vi "Measure Jt curve.vi"(4 "Skip pixel?":bool, 6 "Scan settings":T1={"J-V scan"=TRUE, "J-t scan"=FALSE, "Min voltage (V)"=0.0, "Max voltage (V)"=1.4, "Step (V)"=0.01, "Measurement delay (ms)"=10.0, "1st scan FB-SC"=TRUE, "Inverted structure"=FALSE, "Stabilisation time (s)"=0.0, "Stabilisation mode"=0, "Stabilisation value (V or A) "=0.0, "Step time (s)"=1.0, "Integration time"=0, "Repeat light scans"=FALSE, "Stabilisation in the dark?"=FALSE, "J-t Min (V)"=0.0, "J-t Max (V)"=1.4, "J-t Step (V)"=0.01, "Max. power stabilisation"=FALSE, "J-t 1st scan FB-SC"=TRUE, "J-t Inverted structure"=FALSE, "Max power tracking"=FALSE, "Vmp (V)"=0.7, "Total stabilisation time (s)"=100.0, "J-t best pixel only"=0, "Max power best pixel only"=0, "Vmp from J-V scan"=FALSE, "Intensity dependence"=FALSE, "P dep best pixel only"=0, "External quantum efficiency"=FALSE, "EQE best pixel only"=0, "WL min (nm)"=300.0, "WL max (nm)"=900.0, "WL step (nm)"=5.0, "Wait (ms)"=100.0, "No. of repeat scans"=2.0, "Only repeat for best pixel"=0, "Chopper Freq. min (Hz)"=90.0, "Time Constant min (s)"=2.0, "Stabilisation time step (s)"=1.0, "Illumination conditions"=2, "Scan rate min (V/s)"=0.1, "Scan rate max (V/s)"=1.0, "No. of scan rate steps"=1.0, "Scan rate voltage step priority"=FALSE, "Scan rate measurement delay priority"=FALSE, "J-t Illumination conditions"=0, "Chopper Freq. max (Hz)"=200.0, "No. of freq. steps"=1.0, "Time Constant max (s)"=2.0, "No. of t const. steps"=1.0, "White bias min (no. of suns)"=0.1, "White bias max (no. of suns)"=1.0, "No. of white bias steps"=1.0, "Repeat EQE scans"=FALSE, "No. of EQE scans"=2.0, "Max P stab. Specific voltage"=FALSE} {"No. of EQE scans" min=1.0 step=1.0; "No. of white bias steps" min=1.0 step=1.0; "No. of t const. steps" min=1.0 step=1.0; "Time Constant max (s)" items=["0.01s", "0.03s", "0.1s", "0.3s", "1s", "3s"]; "No. of freq. steps" min=1.0 step=1.0; "J-t Illumination conditions" items=["Light only", "Dark only", "Light then dark", "Dark then light"]; "No. of scan rate steps" min=1.0 step=1.0; "Illumination conditions" items=["Light only", "Dark only", "Light then dark", "Dark then light", "Light then dark then light", "Dark then light then dark"]; "Time Constant min (s)" items=["0.01s", "0.03s", "0.1s", "0.3s", "1s", "3s"]; "Only repeat for best pixel" items=["only for best pixel", "for best 2 pixels", "for best 3 pixels", "for best 4 pixels", "for best 5 pixels", "for best 6 pixels", "for best 7 pixels", "for all pixels"]; "No. of repeat scans" min=1.0 step=1.0; "EQE best pixel only" items=["only the best pixel", "the best 2 pixel", "the best 3 pixel", "the best 4 pixel", "the best 5 pixel", "the best 6 pixel", "the best 7 pixel", "all pixels"]; "P dep best pixel only" items=["only the best pixel", "the best 2 pixels", "the best 3 pixels", "the best 4 pixels", "the best 5 pixels", "the best 6 pixels", "the best 7 pixels", "all pixels"]; "Max power best pixel only" items=["only the best pixel", "the best 2 pixels", "the best 3 pixels", "the best 4 pixels", "the best 5 pixels", "the best 6 pixels", "the best 7 pixels", "all pixels"]; "J-t best pixel only" items=["only the best pixel", "the best 2 pixels", "the best 3 pixels", "the best 4 pixels", "the best 5 pixels", "the best 6 pixels", "the best 7 pixels", "all pixels"]; "Integration time" items=["Fast", "Normal", "High Accuracy"]; "Stabilisation mode" items=["V", "I"]; "Measurement delay (ms)" min=10.0}, 7 "Cell details cluster":T3={"Cell Position"=16, "Cell Label"="", "Pixel to measure"=0, "Area (cm^2)"=0.126, "Variable"="", "Variable value"="", "Scan settings in queue"=0, "Light or dark"="", "Measurement Type"=""} {"Pixel to measure" items=["All", "1", "2", "3", "4", "5", "6", "7", "8"]}, 10 "Experiment Title":string, 11 "User Name":string) -> (3 "Jt Curve":cluster{"Y":dbl[], "Y":dbl[]}[](graph) caption="JV Curve")   [LabVIEW 2011]
uses:
  TypeDefs/Scan settings.ctl
  TypeDefs/Settings Boolean.ctl
  <instrlib>/keithley_24xx/Keithley 24XX/Keithley 24XX.lvlib
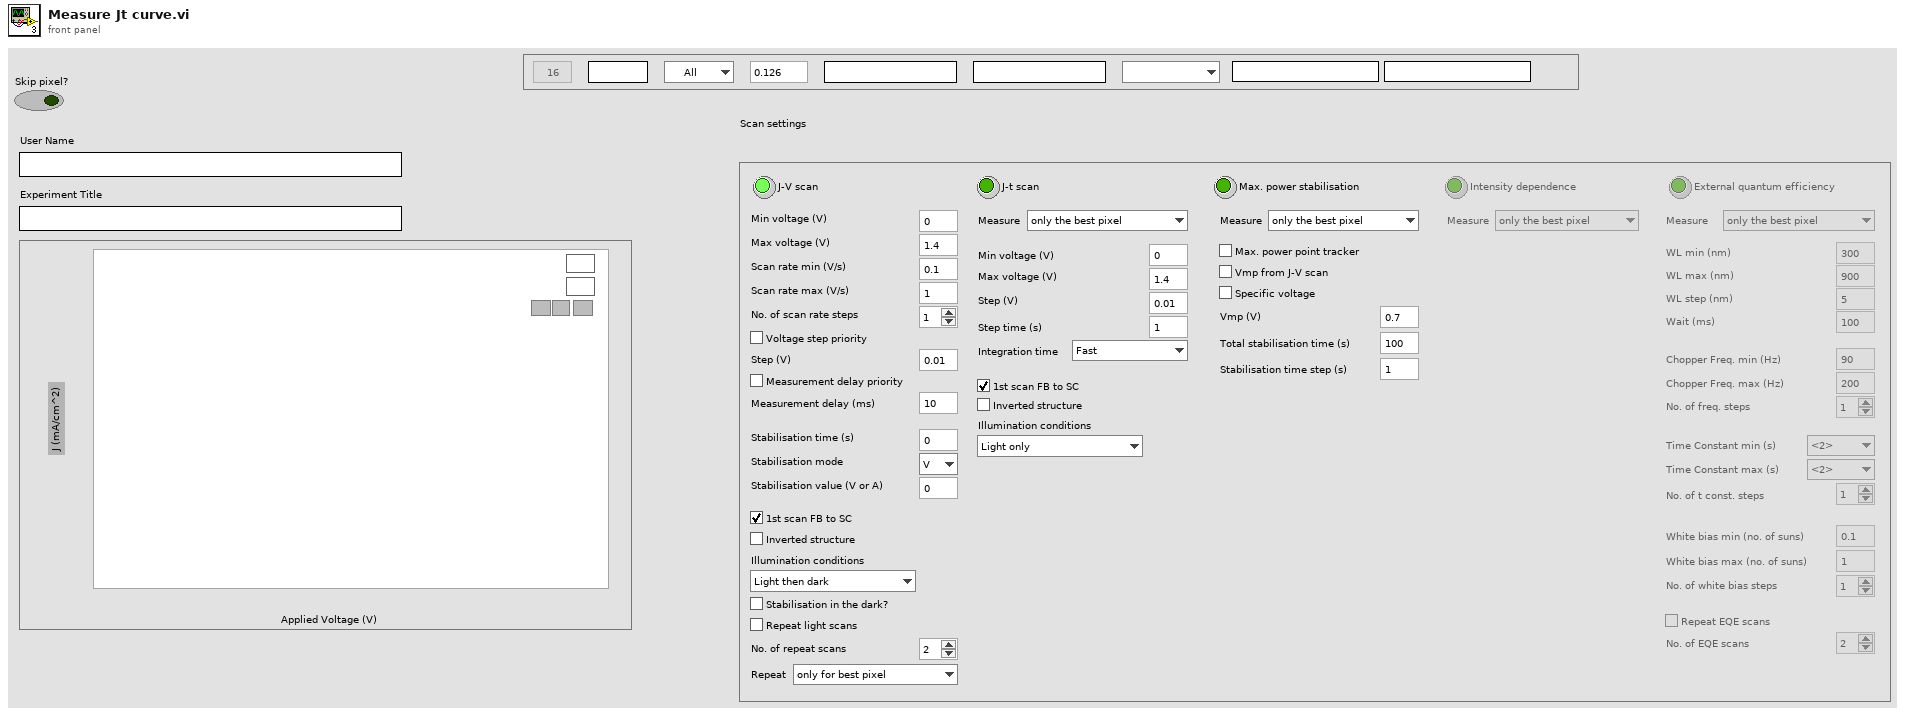
[diagram p1: front panel]
types:
  T1 = typedef "Scan settings.ctl" = cluster{"J-V scan":T2, "J-t scan":bool, "Min voltage (V)":dbl, "Max voltage (V)":dbl, "Step (V)":dbl, "Measurement delay (ms)":dbl, "1st scan FB-SC":bool, "Inverted structure":bool, "Stabilisation time (s)":dbl, "Stabilisation mode":u16, "Stabilisation value (V or A) ":dbl, "Step time (s)":dbl, "Integration time":u16, "Repeat light scans":bool, "Stabilisation in the dark?":bool, "J-t Min (V)":dbl, "J-t Max (V)":dbl, "J-t Step (V)":dbl, "Max. power stabilisation":bool, "J-t 1st scan FB-SC":bool, "J-t Inverted structure":bool, "Max power tracking":bool, "Vmp (V)":dbl, "Total stabilisation time (s)":dbl, "J-t best pixel only":u16, "Max power best pixel only":u16, "Vmp from J-V scan":bool, "Intensity dependence":bool, "P dep best pixel only":u16, "External quantum efficiency":bool, "EQE best pixel only":u16, "WL min (nm)":dbl, "WL max (nm)":dbl, "WL step (nm)":dbl, "Wait (ms)":dbl, "No. of repeat scans":dbl, "Only repeat for best pixel":u16, "Chopper Freq. min (Hz)":dbl, "Time Constant min (s)":dbl, "Stabilisation time step (s)":dbl, "Illumination conditions":u16, "Scan rate min (V/s)":dbl, "Scan rate max (V/s)":dbl, "No. of scan rate steps":dbl, "Scan rate voltage step priority":bool, "Scan rate measurement delay priority":bool, "J-t Illumination conditions":u16, "Chopper Freq. max (Hz)":dbl, "No. of freq. steps":dbl, "Time Constant max (s)":dbl, "No. of t const. steps":dbl, "White bias min (no. of suns)":dbl, "White bias max (no. of suns)":dbl, "No. of white bias steps":dbl, "Repeat EQE scans":bool, "No. of EQE scans":dbl, "Max P stab. Specific voltage":bool}
  T2 = typedef "Settings Boolean.ctl" = bool
  T3 = cluster{"Cell Position":i32, "Cell Label":string, "Pixel to measure":u16, "Area (cm^2)":dbl, "Variable":string, "Variable value":string, "Scan settings in queue":u16, "Light or dark":string, "Measurement Type":string}
  T4 = typedef "imagedata.ctl" = cluster{"image type":i32, "image depth":i32, "image":u8[], "mask":u8[], "colors":u32[], "Rectangle":cluster{"left":i16, "top":i16, "right":i16, "bottom":i16}}
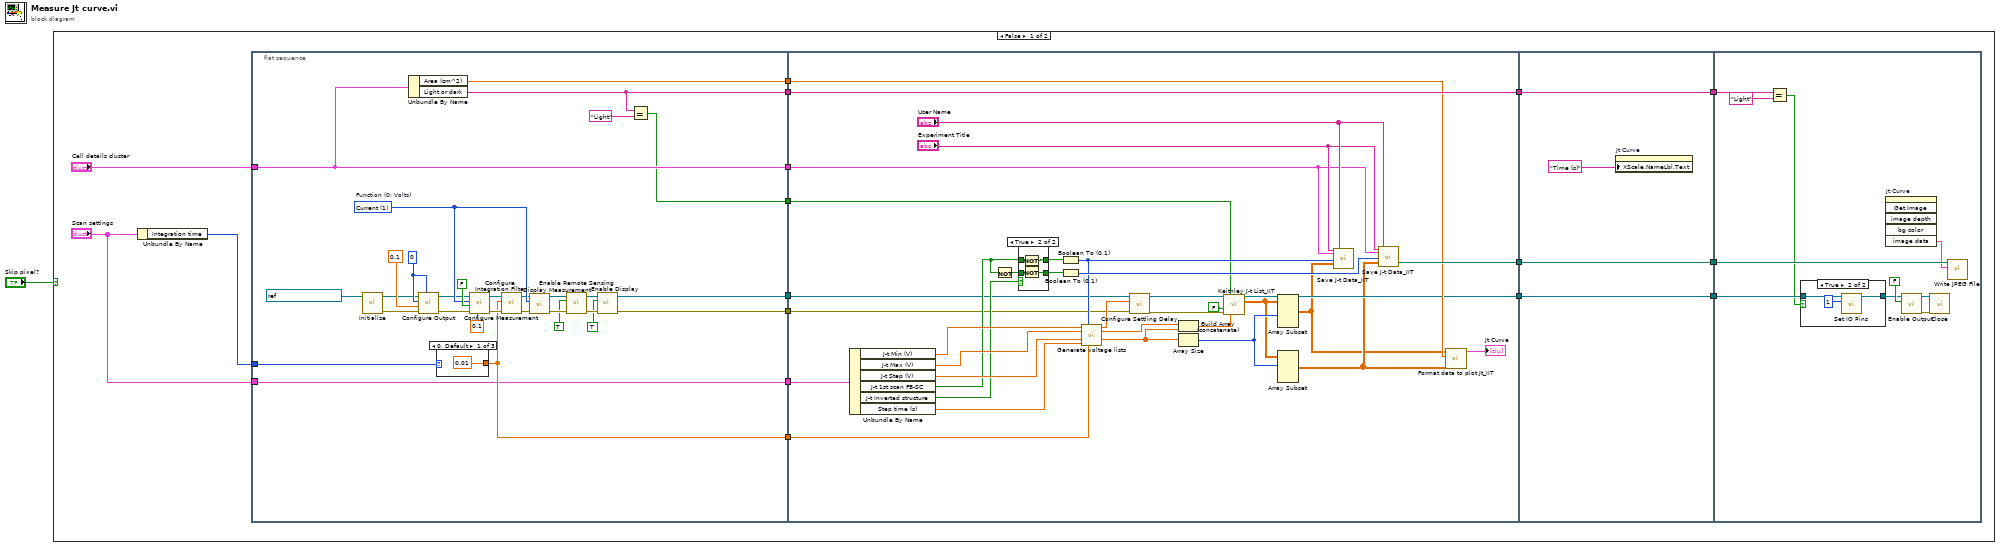
[diagram p0: block diagram]
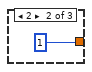
[diagram p2: hidden frame]
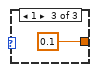
[diagram p3: hidden frame]
diagram:
  n1 = case shown="False" "Skip pixel?" {
    frame False {
      n2 = Unbundle By Name("Scan settings") -> ("Integration time"=w10:u16)
      n3 = flat-sequence {
        tunnel: [w19] -> w17
        tunnel: [w20] -> w18
        tunnel: [w37] -> w16
        tunnel: w10 -> [w36]
        tunnel: [w33] -> w15
        tunnel: "Cell details cluster" -> [w33]
        tunnel: [w35] -> w14
        tunnel: "Scan settings" -> [w35]
        tunnel: [w32] -> w13
        tunnel: [w31] -> w12
        tunnel: [w21] -> w11
        tunnel: [w61] -> w7
        tunnel: [w83] -> w5
        tunnel: w18 -> [w64]
        tunnel: w17 -> [w63]
        tunnel: w16 -> [w80]
        tunnel: w15 -> [w67]
        tunnel: w14 -> [w77]
        tunnel: [w69] -> w3
        tunnel: w13 -> [w69]
        tunnel: w12 -> [w68]
        tunnel: w11 -> [w52]
        tunnel: w7 -> [w96]
        tunnel: [w96] -> w6
        tunnel: w5 -> [w95]
        tunnel: [w95] -> w4
        tunnel: w3 -> [w94]
        tunnel: [w94] -> w2
        tunnel: w6 -> [w100]
        tunnel: w4 -> [w103]
        tunnel: w2 -> [w97]
        frame #0 {
          w26 = 0
          w39 = u16 1 items=["Volts", "Current", "Resistance"]  # Function (0: Volts)
          n4 = call <instrlib>:"Initialize.vi"("VISA resource name"=refnum<visa-resource-name> "GPIB0::24::INSTR") -> ("error out"=w24:errorcluster, "VISA resource name out"=w25:refnum<visa-resource-name>)  [unwired: 4 in, 5 out]
          n5 = Unbundle By Name(w33) -> ("Area (cm^2)"=w31:dbl, "Light or dark"=w32:string)
          n6 = call <instrlib>:"Configure Output.vi"("Source Mode  (0: Voltage)"=w26, "error in (no error)"=w24, "Compliance  Level (0.1)"=0.1, "Output Level (0)"=w26, "VISA resource name"=w25) -> ("error out"=w22:errorcluster, "VISA resource name out"=w23:refnum<visa-resource-name>)  [unwired: 5 in]
          n7 = case shown="0, Default" w36 {
            tunnel: [0.01 1 0.1] -> w37
            frame 0, Default {
            }
            frame 2 {
            }
            frame 1 {
            }
          }
          n8 = call <instrlib>:"Configure Measurement.vi"("Manual Range (1.0)"=0.1, "error in (no error)"=w22, "Enable Auto Range (T:Enable)"=FALSE, "Function (0: Volts)"=w39, "VISA resource name"=w23) -> ("error out"=w44:errorcluster, "VISA resource name out"=w43:refnum<visa-resource-name>)  [unwired: 5 in]
          n9 = call <instrlib>:"Configure Integration Filter.vi"("error in (no error)"=w44, "Measurement Speed (1 PLC)"=w37, "VISA resource name"=w43) -> ("error out"=w29:errorcluster, "VISA resource name out"=w30:refnum<visa-resource-name>)  [unwired: 7 in]
          n10 = call <instrlib>:"Display Measurement.vi"("error in (no error)"=w29, "Displayed Measurement (0: Voltage)"=w39, "VISA resource name"=w30) -> ("error out"=w46:errorcluster, "VISA resource name out"=w45:refnum<visa-resource-name>)  [unwired: 7 in]
          n11 = call <instrlib>:"Enable Remote Sensing.vi"("error in (no error)"=w46, "Enable Remote Sensing (T: Enable)"=TRUE ("Enable Output (T: Enable)"), "VISA resource name"=w45) -> ("error out"=w41:errorcluster, "VISA resource name out"=w42:refnum<visa-resource-name>)  [unwired: 7 in]
          n12 = call <instrlib>:"Enable Display.vi"("error in (no error)"=w41, "Enable Display (T: Enable)"=TRUE ("Enable Output (T: Enable)"), "VISA resource name"=w42) -> ("error out"=w19:errorcluster, "VISA resource name out"=w20:refnum<visa-resource-name>)  [unwired: 7 in]
          n13 = Equal?(x=w32, y="Light") -> (x = y?=w21:bool)
        }
        frame #1 {
          n14 = Unbundle By Name(w77) -> ("J-t Min (V)"=w76:dbl, "J-t Max (V)"=w75:dbl, "J-t Step (V)"=w74:dbl, "J-t 1st scan FB-SC"=w72:bool, "J-t Inverted structure"=w71:bool, "Step time (s)"=w73:dbl)
          n15 = Not(x=w72) -> (.not. x?=w84:bool)
          n16 = case shown="True" w71 {
            tunnel: [w88 w92] -> w86
            tunnel: [w87 w91] -> w85
            tunnel: w84 -> [w87 w90]
            tunnel: w72 -> [w88 w89]
            frame False {
            }
            frame True {
              n17 = Not(x=w89) -> (.not. x?=w92:bool)
              n18 = Not(x=w90) -> (.not. x?=w91:bool)
            }
          }
          n19 = Boolean To (0,1)(Boolean=w86) -> (0, 1=w81:i16)
          n20 = Boolean To (0,1)(Boolean=w85) -> (0, 1=w82:i16)
          n21 = call "Generate voltage lists.vi"("MinVoltage"=w76, "Initial sweep direction"=w81, "Max Voltage"=w75, "V step"=w74, "t step"=w73, "NPLC"=w80) -> ("Meas. delay (s)"=w65:dbl, "Voltage Forward List"=w62:dbl[], "Voltage Reverse List"=w60:dbl[])  [unwired: 7 in]
          n22 = call <instrlib>:"Configure Settling Delay.vi"("error in (no error)"=w63, "Manual Settling Delay (0 sec)"=w65, "VISA resource name"=w64) -> ("error out"=w53:errorcluster, "VISA resource name out"=w55:refnum<visa-resource-name>)  [unwired: 7 in]
          n23 = Build Array (concatenate)(w62, w60) -> (w54:dbl[])
          n24 = Array Size(array=w60) -> (size(s)=w58:i32)
          n25 = call "Keithley J-t List_IIT.vi"("VISA resource name in"=w55, "Shutter open?"=w52, "Light?"=FALSE, "error in (no error)"=w53, "Voltage List"=w54) -> ("VISA resource name out"=w61:refnum<visa-resource-name>, "Data Array"=w57:dbl[][])  [unwired: 7 in, 2 out]
          n26 = Array Subset(array=w57, length (row)=w58) -> (w56:dbl[][])  [unwired: 3 in]
          n27 = Array Subset(array=w57, index (row)=w58) -> (w59:dbl[][])  [unwired: 3 in]
          n28 = call "Save J-t Data_IIT.vi"("Experiment Indicator"="Experiment Title", "Cell details cluster"=w67, "Scan direction"=w81, "Data Array"=w56, "Username"="User Name") -> ()  [unwired: 13 in, 2 out]
          n29 = call "Save J-t Data_IIT.vi"("Experiment Indicator"="Experiment Title", "Cell details cluster"=w67, "Scan direction"=w82, "Data Array"=w59, "Username"="User Name") -> ("File path for JV image"=w83:path)  [unwired: 13 in, 1 out]
          n30 = call "Format data to plot Jt_IIT.vi"("Data Array 2"=w59, "Device Area (cm^2)"=w68, "Data Array"=w56) -> ("JV Curve"=→"Jt Curve":cluster{"Y":dbl[], "Y":dbl[]}[])  [unwired: 8 in]
        }
        frame #2 {
          n31 = property on="Jt Curve" class="XYGraph (strict)"("XScale.NameLbl.Text"="Time (s)" ("Y Scale.Name Label.Text")) -> ()  [unwired: 2 in, 2 out]
        }
        frame #3 {
          n32 = Equal?(x=w97, y="Light") -> (x = y?=w98:bool)
          n33 = case shown="True" w98 {
            tunnel: w100 -> [w107 w109]
            tunnel: [w107 w108] -> w99
            frame False {
            }
            frame True {
              n34 = call <instrlib>:"Set IO Pins.vi"("Output Pattern (0)"=1, "VISA resource name"=w109) -> ("VISA resource name out"=w108:refnum<visa-resource-name>)  [unwired: 8 in, 1 out]
            }
          }
          n35 = invoke on="Jt Curve" class="XYGraph (strict)" method="Get Image"() -> ("image data"=w102:T4)  [unwired: 6 in, 5 out]
          n36 = call <instrlib>:"Enable Output.vi"("Enable Output (T: Enable)"=FALSE ("Output (Off)"), "VISA resource name"=w99) -> ("error out"=w105:errorcluster, "VISA resource name out"=w106:refnum<visa-resource-name>)  [unwired: 8 in]
          n37 = call <instrlib>:"Close.vi"("error in (no error)"=w105, "VISA resource name"=w106) -> ()  [unwired: 9 in, 1 out]
          n38 = call <vilib>:"Write JPEG File.vi"("image data"=w102, "path to JPEG file"=w103) -> ()  [unwired: 8 in, 2 out]
        }
      }
    }
    frame True {
    }
  }
